vi "Drag.vi"(8 "error in (no error)":errorcluster, 10 "DragPosition":i32, 11 "OrderSelection in":refnum<class "OrderSelection.lvclass">) -> (0 "error out":errorcluster, 3 "OrderSelection out":refnum<class "OrderSelection.lvclass">)   [LabVIEW 2020, in "OrderSelection.lvclass"]
uses:
  OrderSelection.lvclass
  C:/Program Files/National Instruments/LabVIEW 2020/vi.lib/QSI/QControls/QControl Classes/Picture/Picture.lvclass
  Read Items.vi
  Read ItemGraphic.vi
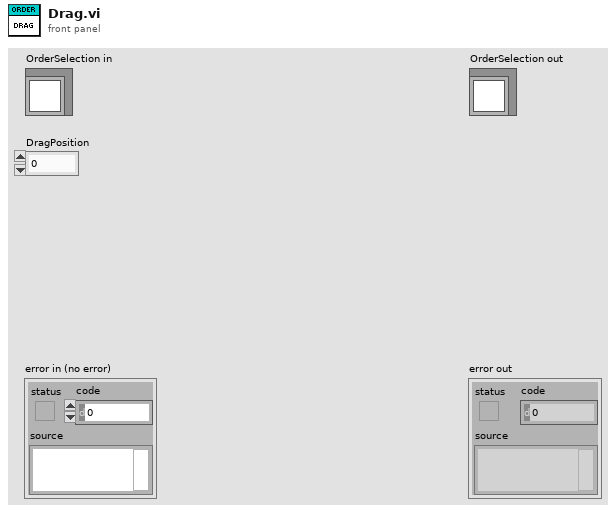
[diagram p1: front panel]
types:
  T1 = typedef "LVBoundsTypeDef.ctl" = cluster{"Width":u32, "Height":u32}
  T2 = typedef "imagedata.ctl" = cluster{"image type":i32, "image depth":i32, "image":u8[], "mask":u8[], "colors":u32[], "Rectangle":cluster{"left":i16, "top":i16, "right":i16, "bottom":i16}}
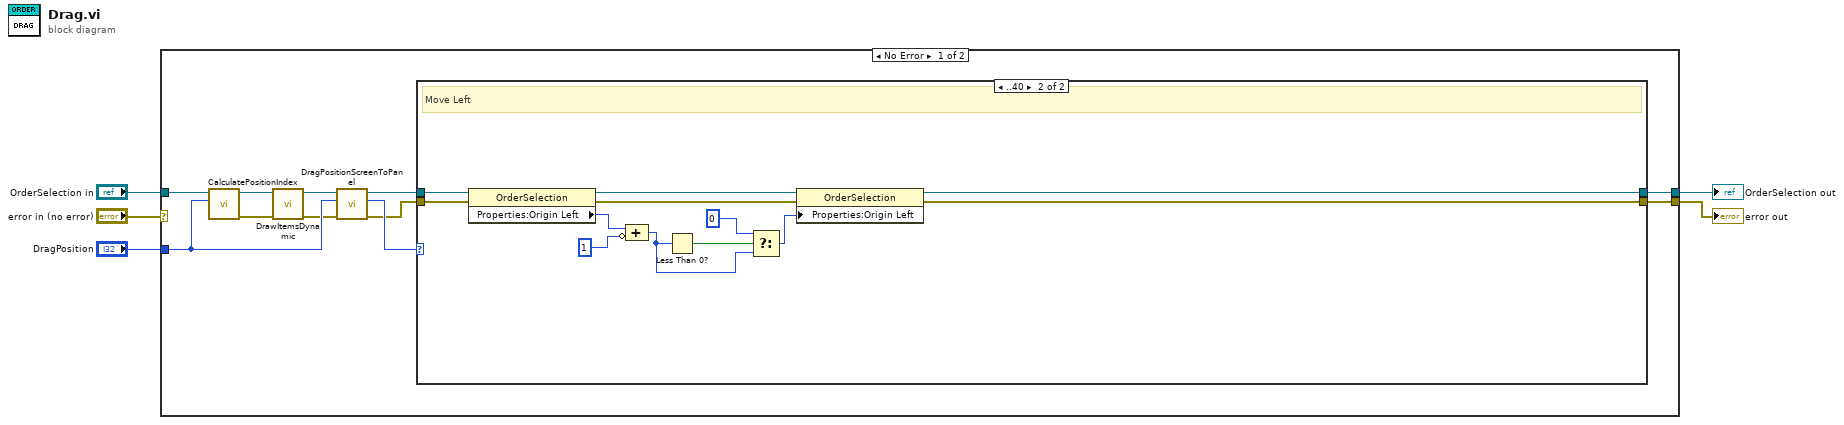
[diagram p0: block diagram]
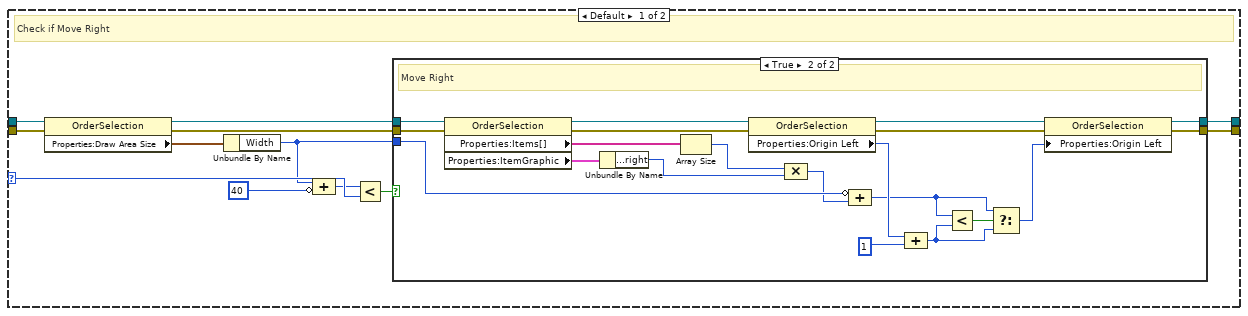
[diagram p2: hidden frame]
diagram:
  n1 = case shown="No Error" "error in (no error)" {
    selector: "error in (no error)" -> [_ w64]
    tunnel: [w16 w64] -> w4
    tunnel: [w15 w63] -> w2
    tunnel: "OrderSelection in" -> [w12 w63]
    tunnel: "DragPosition" -> [w13 _]
    frame No Error {
      n2 = call "CalculatePositionIndex.vi"("DragPosition"=w13, "OrderSelection in"=w12) -> ("error out"=w10:errorcluster, "OrderSelection out"=w11:refnum<class "OrderSelection.lvclass">)  [unwired: 8 in]
      n3 = call "DrawItemsDynamic.vi"("error in (no error)"=w10, "OrderSelection in"=w11) -> ("error out"=w6:errorcluster, "OrderSelection out"=w9:refnum<class "OrderSelection.lvclass">)  [unwired: 8 in]
      n4 = call "DragPositionScreenToPanel.vi"("error in (no error)"=w6, "DragPosition (Screen)"=w13, "OrderSelection in"=w9) -> ("error out"=w7:errorcluster, "DragPosition (Panel)"=w14:i32, "OrderSelection out"=w8:refnum<class "OrderSelection.lvclass">)  [unwired: 6 in]
      n5 = case shown="..40" w14 {
        selector: w14 -> [w26 _]
        tunnel: w7 -> [w20 w62]
        tunnel: [w25 w61] -> w16
        tunnel: w8 -> [w22 w53]
        tunnel: [w27 w60] -> w15
        frame Default {
          # "Check if Move Right"
          n6 = property class="OrderSelection"(reference=w22, error in=w20) -> (reference out=w21:refnum<class "OrderSelection.lvclass">, error out=w19:errorcluster, "Properties:Draw Area Size"=w18:T1)
          n7 = Unbundle By Name(w18) -> ("Width"=w17:u32)
          n8 = Compound Arithmetic op=ADD(w17, invert u32 40 ("value")) -> (w23:u32)
          n9 = Less?(x=w23, y=w26) -> (x < y?=w28:bool)
          n10 = case shown="True" w28 {
            tunnel: w21 -> [w30 w38]
            tunnel: [w30 w48] -> w27
            tunnel: w19 -> [w29 w35]
            tunnel: [w29 w47] -> w25
            tunnel: w17 -> [_ w41]
            frame False {
              # "Do Nothing"
            }
            frame True {
              # "Move Right"
              n11 = property class="OrderSelection"(reference=w38, error in=w35) -> (reference out=w37:refnum<class "OrderSelection.lvclass">, error out=w36:errorcluster, "Properties:Items[]"=w34:string[], "Properties:ItemGraphic"=w32:T2)
              n12 = Unbundle By Name(w32) -> ("Rectangle.right"=w31:i16)
              n13 = Array Size(array=w34) -> (size(s)=w33:i32)
              n14 = property class="OrderSelection"(reference=w37, error in=w36) -> (reference out=w43:refnum<class "OrderSelection.lvclass">, error out=w44:errorcluster, "Properties:Origin Left"=w42:i16)
              n15 = Compound Arithmetic op=MULTIPLY(w33, w31) -> (w39:i32)
              n16 = Compound Arithmetic op=ADD(invert w41, w39) -> (w40:u32)
              n17 = Compound Arithmetic op=ADD(w42, i16 1 ("value")) -> (w45:i16)
              n18 = Less?(x=w40, y=w45) -> (x < y?=w46:bool)
              n19 = Select(t=w40, s=w46, f=w45) -> (s? t:f=w50:u32)
              n20 = property class="OrderSelection"(reference=w43, error in=w44, "Properties:Origin Left"=w50) -> (reference out=w48:refnum<class "OrderSelection.lvclass">, error out=w47:errorcluster)
            }
          }
        }
        frame ..40 {
          # "Move Left"
          n21 = property class="OrderSelection"(reference=w53, error in=w62) -> (reference out=w52:refnum<class "OrderSelection.lvclass">, error out=w54:errorcluster, "Properties:Origin Left"=w51:i16)
          n22 = Compound Arithmetic op=ADD(w51, invert i16 1 ("value")) -> (w56:i16)
          n23 = Less Than 0?(x=w56) -> (x < 0?=w59:bool)
          n24 = Select(t=i16 0, s=w59, f=w56) -> (s? t:f=w57:i16)
          n25 = property class="OrderSelection"(reference=w52, error in=w54, "Properties:Origin Left"=w57) -> (reference out=w60:refnum<class "OrderSelection.lvclass">, error out=w61:errorcluster)
        }
      }
    }
    frame Error {
    }
  }
  "error out" <- w4
  "OrderSelection out" <- w2
